vi "read_data.vi"(8 "error in (no error)":errorcluster, 11 "StreamingBase in":refnum<class "StreamingBase.lvclass">) -> (0 "error out":errorcluster, 2 "data variants":variant[](array[variant]), 3 "StreamingBase out":refnum<class "StreamingBase.lvclass">)   [LabVIEW 2011, in "StreamingBase.lvclass"]
uses:
  StreamingBase.lvclass
  StreamingBase.lvclass/StreamingBase.ctl
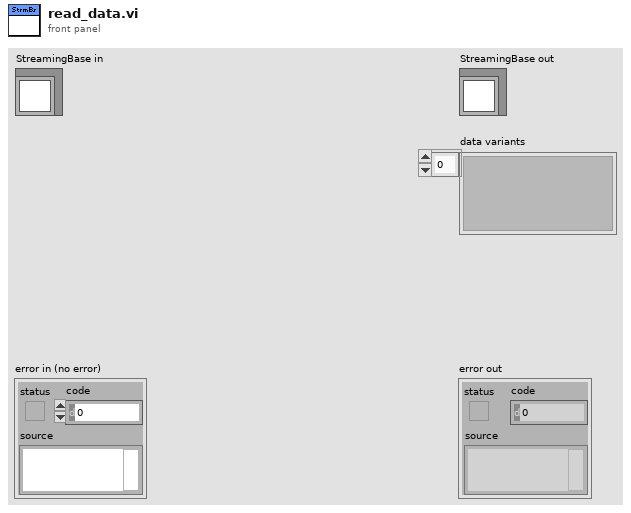
[diagram p1: front panel]
types:
  T1 = typedef "StreamingBase.lvclass/observer_cluster.ctl" = cluster{"writer endpoint":refnum<k21>, "reader endpoint":refnum<k21>, "wait for response?":bool}
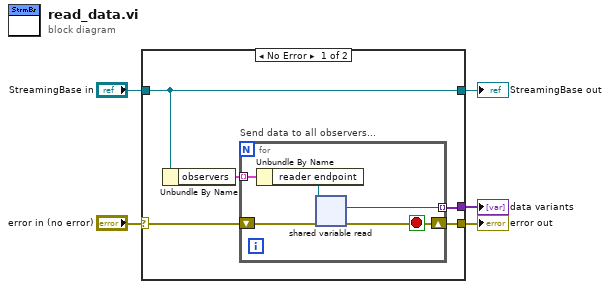
[diagram p0: block diagram]
diagram:
  n1 = case shown="No Error" "error in (no error)" {
    selector: "error in (no error)" -> [w9 w17]
    tunnel: [w8 w17] -> w4
    tunnel: [w6 w16] -> w2
    tunnel: "StreamingBase in" -> [w6 w16]
    tunnel: [w7 _] -> w1
    frame No Error {
      n2 = Unbundle By Name(w6) -> ("observers"=w10:T1[])
      n3 = for "Send data to all observers..." {
        shift-right: [w12] -> w8
        shift-left: w9 -> [w13]
        tunnel: w10 -> [w15] mode=indexing
        tunnel: [w11] -> w7 mode=indexing
        stop <- w12 stop-if-true
        n4 = Unbundle By Name(w15) -> ("reader endpoint"=w14:refnum<k21>)
        n5 = shared-variable-read(w14, w13) -> (w12:errorcluster, w11:variant)  [unwired: 1 in, 2 out]
      }
    }
    frame Error {
    }
  }
  "error out" <- w4
  "StreamingBase out" <- w2
  "data variants" <- w1
